vi "Read_Event_Arduino.vi"(8 "error in":errorcluster, 9 "condition":i32, 10 "Progress in":u8=50, 11 "VISA resource name in":refnum<visa-resource-name>) -> (0 "error out":errorcluster, 1 "Progress":u8, 2 "output":i32, 3 "VISA resource name out":refnum<visa-resource-name>)   [LabVIEW 2018]
panel:
  out "concatenated string":string
  out "Serial Settings:Number of Bytes at Serial Port":u32
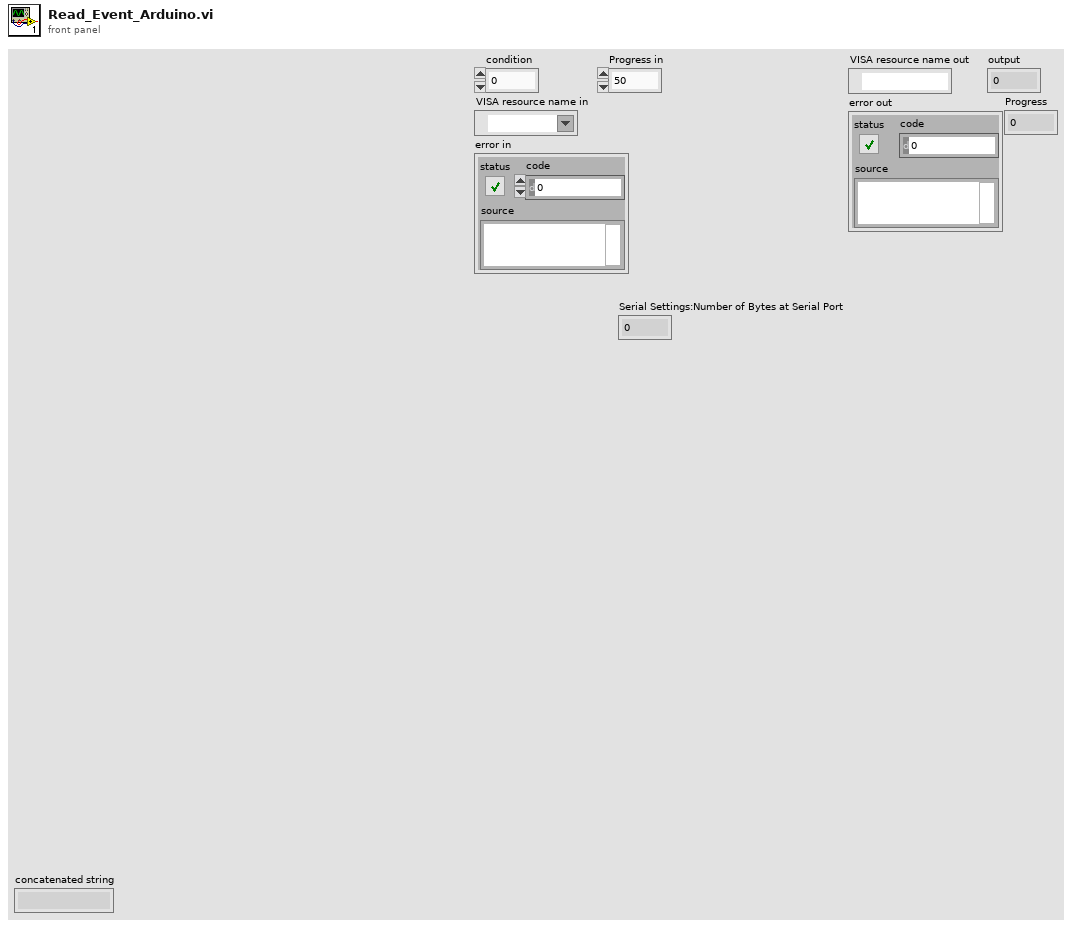
[diagram p1: front panel]
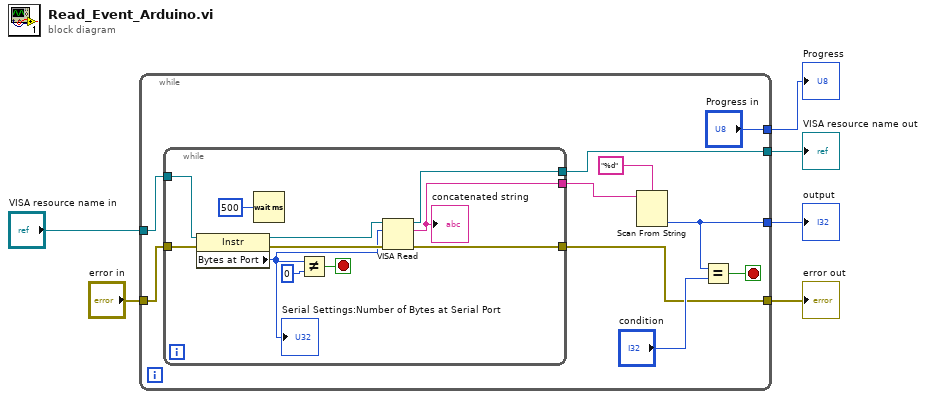
[diagram p0: block diagram]
diagram:
  n1 = while {
    tunnel: ["Progress in"] -> w5
    tunnel: [w13] -> w6
    tunnel: "VISA resource name in" -> [w11]
    tunnel: "error in" -> [w10]
    tunnel: [w9] -> w2
    tunnel: [w8] -> w1
    stop <- w15 stop-if-true
    n2 = while {
      tunnel: [w25] -> w8
      tunnel: [w24] -> w9
      tunnel: [w20] -> w7
      tunnel: w11 -> [w19]
      tunnel: w10 -> [w18]
      stop <- w26 stop-if-true
      n3 = property class="Instr"(reference=w19, error in=w18) -> (reference out=w23:refnum<visa-resource-name>, error out=w22:errorcluster, "Bytes at Port"=w21:u32)
      "Serial Settings:Number of Bytes at Serial Port" <- w21
      n4 = Wait (ms)(milliseconds to wait=u32 500) -> ()  [unwired: 1 out]
      n5 = Not Equal?(x=w21, y=0) -> (x != y?=w26:bool)
      n6 = VISA Read(VISA resource name=w23, byte count=w21, error in (no error)=w22) -> (VISA resource name out=w24:refnum<visa-resource-name>, read buffer=w20:string, error out=w25:errorcluster)  [unwired: 1 out]
      "concatenated string" <- w20
    }
    n7 = Scan From String(format string="%d", input string=w7) -> (output 1=w13:i32)  [unwired: 3 in, 3 out]
    n8 = Equal?(x=w13, y="condition") -> (x = y?=w15:bool)
  }
  "VISA resource name out" <- w2
  "error out" <- w1
  "output" <- w6
  "Progress" <- w5
